vi "SUB_CAL_TESTTIME.vi"(3 "Test Item name":string, 4 "Stop tick time":u32, 5 "Start tick time":u32) -> (1 "Test Time output":string)   [LabVIEW 2011]
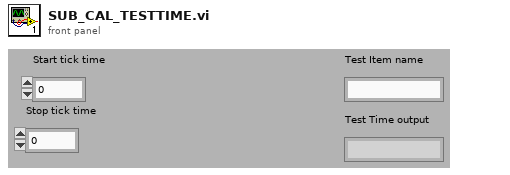
[diagram p1: front panel]
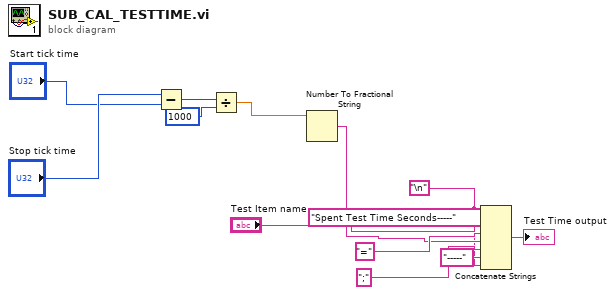
[diagram p0: block diagram]
diagram:
  w4 = "\n"
  n1 = Subtract(x="Stop tick time", y="Start tick time") -> (x-y=w13:u32)
  n2 = Divide(x=w13, y=u32 1000) -> (x/y=w1:dbl)
  n3 = Number To Fractional String(number=w1) -> (F-format string=w8:string)  [unwired: 3 in]
  n4 = Concatenate Strings(w4, "Spent Test Time Seconds-----" ("string"), "Test Item name", "=", w8, ";", "-----" ("string"), w4) -> (→"Test Time output":string)
